vi "PH_PP_CurrentMeas_Test.vi"() -> ()   [LabVIEW 2014, in "PH_PP_CurrentMeas.lvlib"]
doc: "This VI was developed to test the PH_PPMA_DAQ RT Server Application.\n\nPlease use the PH_PPMA_DAQClient Class within the CS framework."
uses:
  PH_PP_CurrentMeas.lvlib
  PH_PP_CurrentMeas.CommandCluster.ctl
panel:
  out "Error unpacking Data? Port 6343":bool
  out "Error unpacking Data? Port 6342":bool
  out "Error unpacking Data? Port 6341":bool
  in  "Reset Error":bool
  out "6343 not connected?":bool
  out "6342 not connected?":bool
  out "6341 not connected?":bool
  out "error out":errorcluster
  in  "Tab Control":enum32{"Port 6341", "Port 6342", "Port 6343"}(tab)
  out "No Connection on 6341":bool
  out "No Data achieved due to \nno Trigger Signal on 6341":bool
  out "No Data achieved due to \nTask Failure on 6341":bool
  out "No Task defined on 6341":bool
  out "Measurement Port 6341":waveform(dbl)[](graph) caption="Measurement Data Port 6341"
  in  "Port 6341":bool
  in  "Check Port 6341":bool
  out "Received Data Sets Port 6341":T1[](array[typedef])
  out "No Connection on 6342":bool
  out "No Data achieved due to \nno Trigger Signal on 6342":bool
  out "No Data achieved due to \nTask Failure on 6342":bool
  out "No Task defined on 6342":bool
  in  "Port 6342":bool
  in  "Check Port 6342":bool
  out "Received Data Sets Port 6342":T1[](array[typedef])
  out "Measurement Port 6342":waveform(dbl)[](graph) caption="Measurement Data Port 6342"
  out "No Connection on 6343":bool
  out "No Data achieved due to \nno Trigger Signal on 6343":bool
  out "No Data achieved due to \nTask Failure on 6343":bool
  out "No Task defined on 6343":bool
  in  "Port 6343":bool
  in  "Check Port 6343":bool
  out "Received Data Sets Port 6343":T1[](array[typedef])
  out "Measurement Port 6343":waveform(dbl)[](graph) caption="Measurement Data Port 6341"
  in  "stop":bool
  in  "DAQ Server":string="phpxi001.gsi.de"
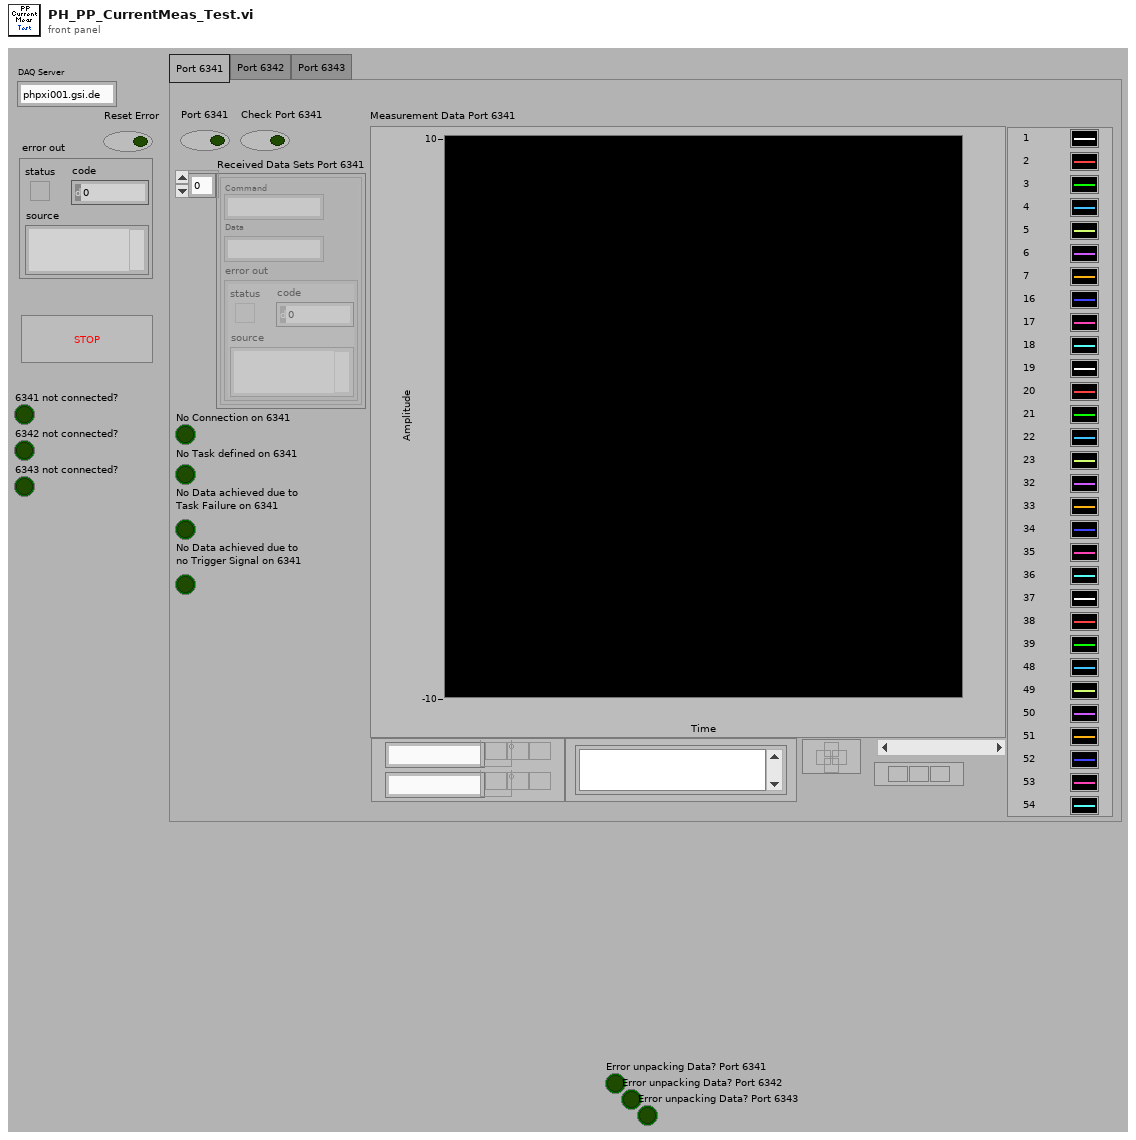
[diagram p1: front panel]
types:
  T1 = typedef "PH_PP_CurrentMeas.lvlib/PH_PP_CurrentMeas.CommandCluster.ctl" = cluster{"Command":string, "Data":string, "error out":errorcluster}
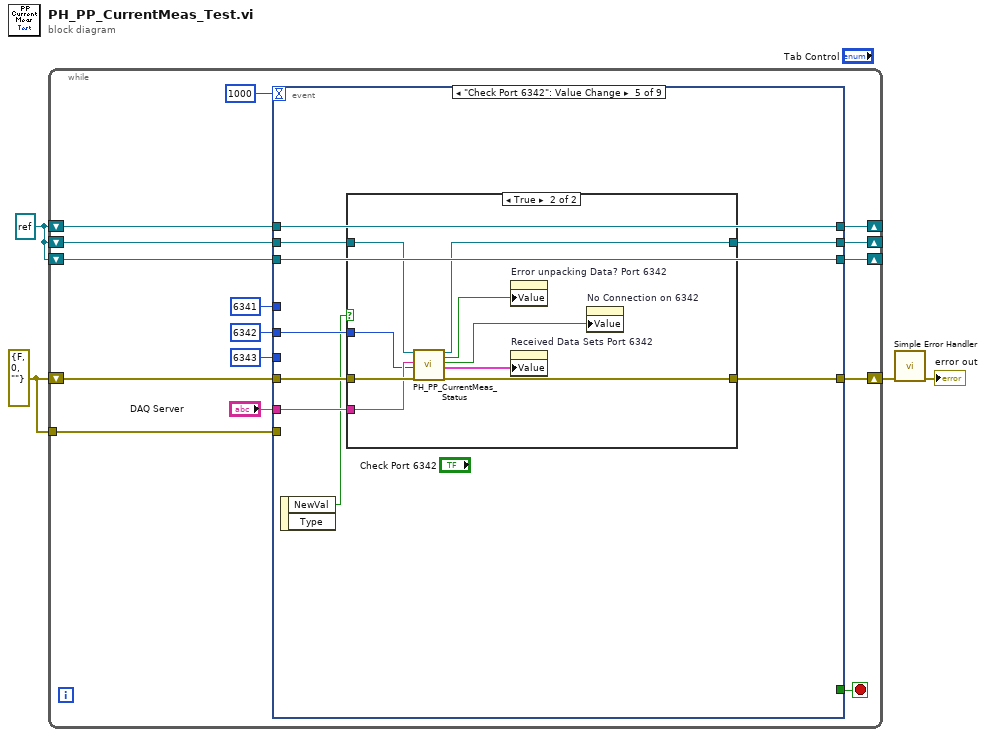
[diagram p0: block diagram]
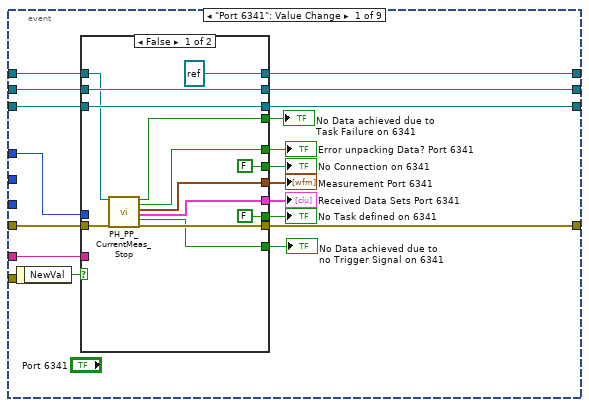
[diagram p2: hidden frame]
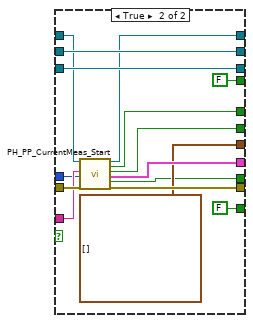
[diagram p3: hidden frame]
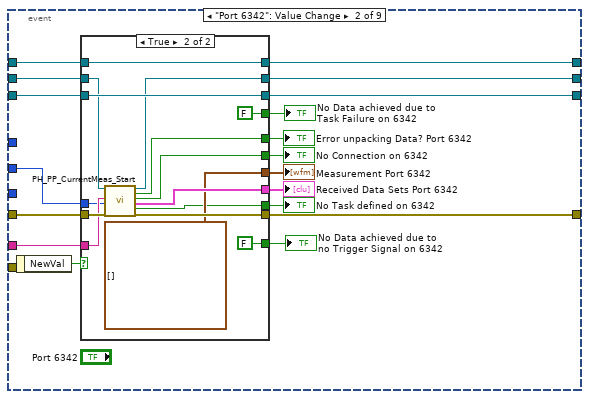
[diagram p4: hidden frame]
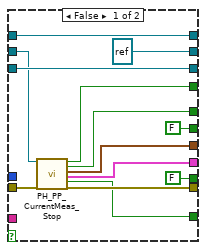
[diagram p5: hidden frame]
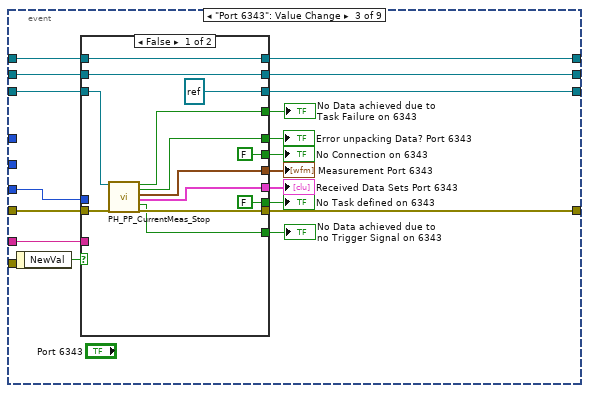
[diagram p6: hidden frame]
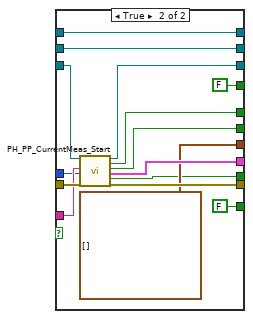
[diagram p7: hidden frame]
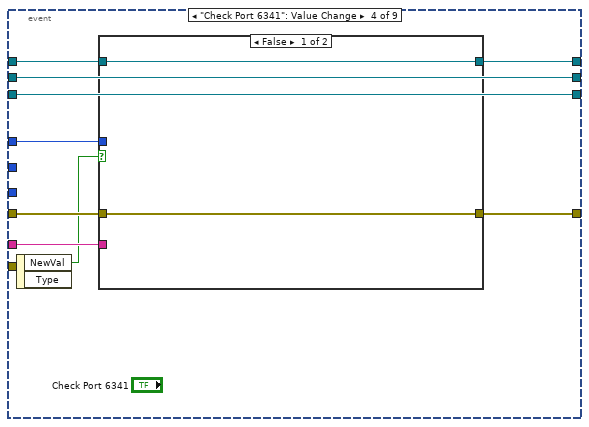
[diagram p8: hidden frame]
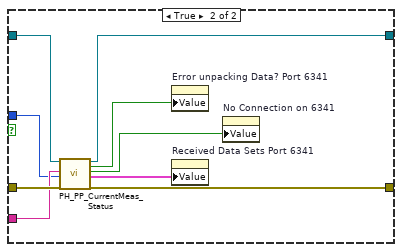
[diagram p9: hidden frame]
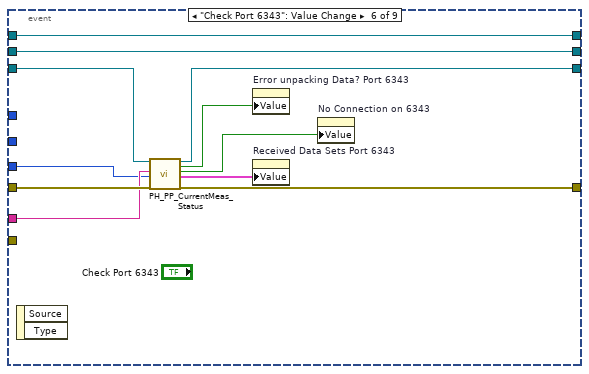
[diagram p11: hidden frame]
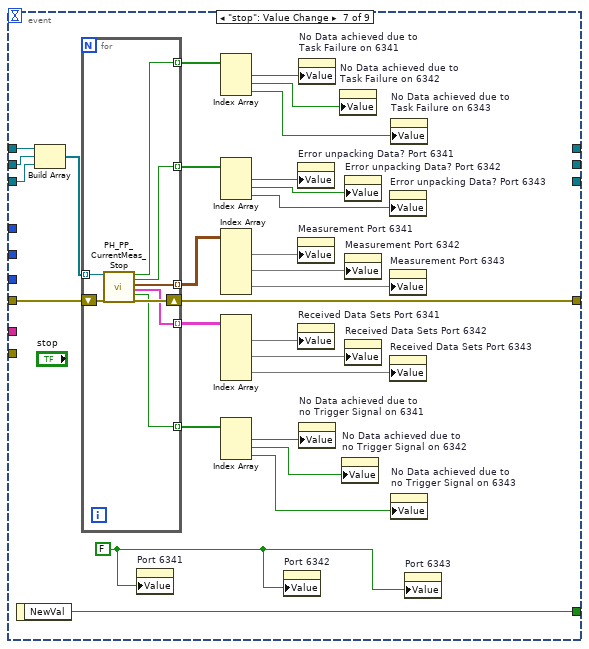
[diagram p12: hidden frame]
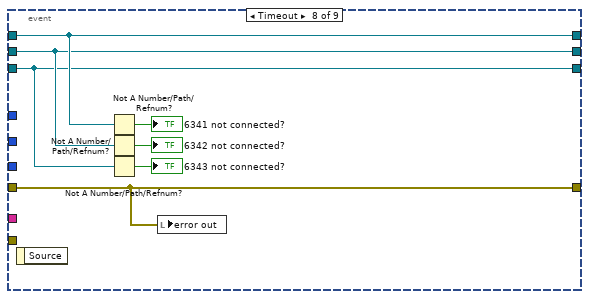
[diagram p13: hidden frame]
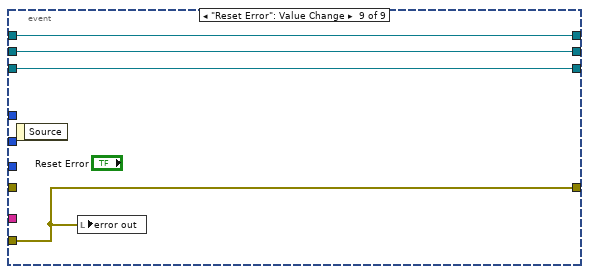
[diagram p14: hidden frame]
diagram:
  w2 = refnum<k5> refnum ("TCP Network Connection out")
  w1 = errorcluster {"status"=FALSE, "code"=0, "source"=""} ("error out")
  n1 = while {
    shift-right: [w12] -> _
    shift-left: w2 -> [w19]
    shift-right: [w16] -> w4
    shift-left: w1 -> [w18]
    shift-right: [w11] -> _
    shift-left: w2 -> [w14]
    shift-right: [w10] -> _
    shift-left: w2 -> [w13]
    tunnel: w1 -> [w5]
    stop <- w17 stop-if-true
    n2 = event shown="[4] \"Check Port 6342\": Value Change" {
      selector: _ -> [_ _ _ _ _ _ _ _ _]
      dyn-events: _ -> [_ _ _ _ _ _ _ _ _]
      timeout: 1000 -> [_ _ _ _ _ _ _ _ _]
      tunnel: w19 -> [w37 w83 w129 w164 w181 w205 w232 w248 w255]
      tunnel: [w36 w82 w128 w163 w181 w205 _ w248 w255] -> w12
      tunnel: [w28 w74 w120 w161 w184 w207 w235 w245 w252] -> w16
      tunnel: w18 -> [w31 w77 w123 w162 w185 w208 w230 w245 _]
      tunnel: [_ _ _ _ _ _ w236 _ _] -> w17
      tunnel: "DAQ Server" -> [w29 w75 w121 w160 w183 w206 _ _ _]
      tunnel: [w34 w80 w126 w166 w179 w203 _ w247 w254] -> w11
      tunnel: w14 -> [w35 w81 w127 w166 w180 w203 w234 w247 w254]
      tunnel: [w32 w78 w124 w165 w186 w201 _ w246 w253] -> w10
      tunnel: w13 -> [w33 w79 w125 w165 w186 w202 w233 w246 w253]
      tunnel: u16 6341 ("Port") -> [w27 _ _ w159 _ _ _ _ _]
      tunnel: u16 6342 ("Port") -> [_ w70 _ _ w182 _ _ _ _]
      tunnel: u16 6343 ("Port") -> [_ _ w116 _ _ w204 _ _ _]
      tunnel: w5 -> [_ _ _ _ _ _ _ _ w252]
      event "Port 6341": Value Change {
        n3 = event-data() -> ("NewVal"=w30:bool)  [unwired: 1 in]
        n4 = case shown="False" w30 {
          tunnel: [refnum<k5> refnum ("connection ID out") w59] -> w36
          tunnel: w37 -> [w46 w60]
          tunnel: [w47 w58] -> w28
          tunnel: w31 -> [w48 w63]
          tunnel: w29 -> [_ w62]
          tunnel: w35 -> [w50 w65]
          tunnel: [w50 w65] -> w34
          tunnel: [w49 w64] -> w32
          tunnel: w33 -> [w49 w64]
          tunnel: w27 -> [_ w61]
          tunnel: [w45 w56] -> w26
          tunnel: [w44 w57] -> w25
          tunnel: [w42 waveform(dbl)[] [] ("Measurement Data")] -> w24
          tunnel: [FALSE ("No Task defined?") w54] -> w23
          tunnel: [FALSE ("Connection not established") w53] -> w22
          tunnel: [w39 FALSE ("No Data achieved due to Task Failure")] -> w21
          tunnel: [w38 FALSE ("No Data achieved due to no Trigger Signal")] -> w20
          frame False {
            n5 = call "PH_PP_CurrentMeas_Stop.vi"("connection ID in"=w46, "error in (no error)"=w48) -> ("No Data achieved due to Task Failure"=w39:bool, "Error unpacking Data?"=w44:bool, "Measurement Data"=w42:waveform(dbl)[], "Receveived Data Sets"=w45:T1[], "No Data achieved due to no Trigger Signal"=w38:bool, "error out"=w47:errorcluster)  [unwired: 12 in]
          }
          frame True {
            n6 = call "PH_PP_CurrentMeas_Start.vi"("connection ID in"=w60, "NI6071E DAQ Server"=w62, "Port"=w61, "error in (no error)"=w63) -> ("connection ID out"=w59:refnum<k5>, "Error unpacking the Data?"=w57:bool, "Connection not established"=w53:bool, "Received Data Sets"=w56:T1[], "No Task defined?"=w54:bool, "error out"=w58:errorcluster)  [unwired: 10 in]
          }
        }
        "Received Data Sets Port 6341" <- w26
        "Error unpacking Data? Port 6341" <- w25
        "Measurement Port 6341" <- w24
        "No Task defined on 6341" <- w23
        "No Connection on 6341" <- w22
        "No Data achieved due to \nTask Failure on 6341" <- w21
        "No Data achieved due to \nno Trigger Signal on 6341" <- w20
      }
      event "Port 6342": Value Change {
        n7 = event-data() -> ("NewVal"=w76:bool)  [unwired: 1 in]
        n8 = case shown="True" w76 {
          tunnel: [w88 w103] -> w82
          tunnel: w83 -> [w88 w103]
          tunnel: [w94 w107] -> w74
          tunnel: w77 -> [w95 w110]
          tunnel: w75 -> [_ w109]
          tunnel: w81 -> [w89 w102]
          tunnel: [refnum<k5> refnum ("connection ID out") w101] -> w80
          tunnel: [w96 w111] -> w78
          tunnel: w79 -> [w96 w111]
          tunnel: w70 -> [_ w108]
          tunnel: [w93 w105] -> w73
          tunnel: [w92 w106] -> w72
          tunnel: [w91 waveform(dbl)[] [] ("Measurement Data")] -> w71
          tunnel: [FALSE ("No Task defined?") w100] -> w69
          tunnel: [FALSE ("Connection not established") w99] -> w68
          tunnel: [w85 FALSE ("No Data achieved due to Task Failure")] -> w67
          tunnel: [w84 FALSE ("No Data achieved due to no Trigger Signal")] -> w66
          frame False {
            n9 = call "PH_PP_CurrentMeas_Stop.vi"("connection ID in"=w89, "error in (no error)"=w95) -> ("No Data achieved due to Task Failure"=w85:bool, "Error unpacking Data?"=w92:bool, "Measurement Data"=w91:waveform(dbl)[], "Receveived Data Sets"=w93:T1[], "No Data achieved due to no Trigger Signal"=w84:bool, "error out"=w94:errorcluster)  [unwired: 12 in]
          }
          frame True {
            n10 = call "PH_PP_CurrentMeas_Start.vi"("connection ID in"=w102, "NI6071E DAQ Server"=w109, "Port"=w108, "error in (no error)"=w110) -> ("connection ID out"=w101:refnum<k5>, "Error unpacking the Data?"=w106:bool, "Connection not established"=w99:bool, "Received Data Sets"=w105:T1[], "No Task defined?"=w100:bool, "error out"=w107:errorcluster)  [unwired: 10 in]
          }
        }
        "Received Data Sets Port 6342" <- w73
        "Error unpacking Data? Port 6342" <- w72
        "Measurement Port 6342" <- w71
        "No Task defined on 6342" <- w69
        "No Connection on 6342" <- w68
        "No Data achieved due to \nTask Failure on 6342" <- w67
        "No Data achieved due to \nno Trigger Signal on 6342" <- w66
      }
      event "Port 6343": Value Change {
        n11 = event-data() -> ("NewVal"=w122:bool)  [unwired: 1 in]
        n12 = case shown="False" w122 {
          tunnel: [w137 w150] -> w128
          tunnel: w129 -> [w137 w150]
          tunnel: [w141 w154] -> w120
          tunnel: w123 -> [w142 w157]
          tunnel: w121 -> [_ w156]
          tunnel: w127 -> [w135 w149]
          tunnel: [w135 w149] -> w126
          tunnel: [refnum<k5> refnum ("connection ID out") w147] -> w124
          tunnel: w125 -> [w134 w148]
          tunnel: w116 -> [_ w155]
          tunnel: [w140 w152] -> w119
          tunnel: [w139 w153] -> w118
          tunnel: [w138 waveform(dbl)[] [] ("Measurement Data")] -> w117
          tunnel: [FALSE ("No Task defined?") w146] -> w115
          tunnel: [FALSE ("Connection not established") w145] -> w114
          tunnel: [w131 FALSE ("No Data achieved due to Task Failure")] -> w113
          tunnel: [w130 FALSE ("No Data achieved due to no Trigger Signal")] -> w112
          frame False {
            n13 = call "PH_PP_CurrentMeas_Stop.vi"("connection ID in"=w134, "error in (no error)"=w142) -> ("No Data achieved due to Task Failure"=w131:bool, "Error unpacking Data?"=w139:bool, "Measurement Data"=w138:waveform(dbl)[], "Receveived Data Sets"=w140:T1[], "No Data achieved due to no Trigger Signal"=w130:bool, "error out"=w141:errorcluster)  [unwired: 12 in]
          }
          frame True {
            n14 = call "PH_PP_CurrentMeas_Start.vi"("connection ID in"=w148, "NI6071E DAQ Server"=w156, "Port"=w155, "error in (no error)"=w157) -> ("connection ID out"=w147:refnum<k5>, "Error unpacking the Data?"=w153:bool, "Connection not established"=w145:bool, "Received Data Sets"=w152:T1[], "No Task defined?"=w146:bool, "error out"=w154:errorcluster)  [unwired: 10 in]
          }
        }
        "Received Data Sets Port 6343" <- w119
        "Error unpacking Data? Port 6343" <- w118
        "Measurement Port 6343" <- w117
        "No Task defined on 6343" <- w115
        "No Connection on 6343" <- w114
        "No Data achieved due to \nno Trigger Signal on 6343" <- w112
        "No Data achieved due to \nTask Failure on 6343" <- w113
      }
      event "Check Port 6341": Value Change {
        n15 = event-data() -> ("NewVal"=w158:bool)  [unwired: 1 in, 1 out]
        n16 = case shown="False" w158 {
          tunnel: w164 -> [w168 w177]
          tunnel: [w168 w176] -> w163
          tunnel: w162 -> [w167 w175]
          tunnel: [w167 w174] -> w161
          tunnel: w160 -> [_ w173]
          tunnel: w159 -> [_ w172]
          frame False {
          }
          frame True {
            n17 = call "PH_PP_CurrentMeas_Status.vi"("connection ID in"=w177, "NI6071E DAQ Server"=w173, "Port"=w172, "error in (no error)"=w175) -> ("connection ID out"=w176:refnum<k5>, "Error unpacking Data?"=w171:bool, "Connection not established"=w169:bool, "Receveived Data Sets"=w170:T1[], "error out"=w174:errorcluster)  [unwired: 11 in]
            n18 = property on="Error unpacking Data? Port 6341" class="Bool (strict)"("Value"=w171) -> ()  [unwired: 2 in, 2 out]
            n19 = property on="Received Data Sets Port 6341" class="Arr (strict)"("Value"=w170) -> ()  [unwired: 2 in, 2 out]
            n20 = property on="No Connection on 6341" class="Bool (strict)"("Value"=w169) -> ()  [unwired: 2 in, 2 out]
          }
        }
      }
      event "Check Port 6342": Value Change {
        n21 = event-data() -> ("NewVal"=w178:bool)  [unwired: 1 in, 1 out]
        n22 = case shown="True" w178 {
          tunnel: w185 -> [w187 w197]
          tunnel: [w187 w196] -> w184
          tunnel: w183 -> [_ w195]
          tunnel: w182 -> [_ w194]
          tunnel: w180 -> [w188 w193]
          tunnel: [w188 w192] -> w179
          frame False {
          }
          frame True {
            n23 = call "PH_PP_CurrentMeas_Status.vi"("connection ID in"=w193, "NI6071E DAQ Server"=w195, "Port"=w194, "error in (no error)"=w197) -> ("connection ID out"=w192:refnum<k5>, "Error unpacking Data?"=w190:bool, "Connection not established"=w189:bool, "Receveived Data Sets"=w191:T1[], "error out"=w196:errorcluster)  [unwired: 11 in]
            n24 = property on="Error unpacking Data? Port 6342" class="Bool (strict)"("Value"=w190) -> ()  [unwired: 2 in, 2 out]
            n25 = property on="Received Data Sets Port 6342" class="Arr (strict)"("Value"=w191) -> ()  [unwired: 2 in, 2 out]
            n26 = property on="No Connection on 6342" class="Bool (strict)"("Value"=w189) -> ()  [unwired: 2 in, 2 out]
          }
        }
      }
      event "Check Port 6343": Value Change {
        n27 = event-data() -> ()  [unwired: 1 in, 2 out]
        n28 = call "PH_PP_CurrentMeas_Status.vi"("connection ID in"=w202, "NI6071E DAQ Server"=w206, "Port"=w204, "error in (no error)"=w208) -> ("connection ID out"=w201:refnum<k5>, "Error unpacking Data?"=w200:bool, "Connection not established"=w198:bool, "Receveived Data Sets"=w199:T1[], "error out"=w207:errorcluster)  [unwired: 11 in]
        n29 = property on="Error unpacking Data? Port 6343" class="Bool (strict)"("Value"=w200) -> ()  [unwired: 2 in, 2 out]
        n30 = property on="Received Data Sets Port 6343" class="Arr (strict)"("Value"=w199) -> ()  [unwired: 2 in, 2 out]
        n31 = property on="No Connection on 6343" class="Bool (strict)"("Value"=w198) -> ()  [unwired: 2 in, 2 out]
      }
      event "stop": Value Change {
        w217 = FALSE
        n32 = event-data() -> ("NewVal"=w236:bool)  [unwired: 1 in]
        n33 = Build Array(w232, w234, w233) -> (w231:refnum<k5>[])
        n34 = for {
          shift-right: [w242] -> w235
          shift-left: w230 -> [w244]
          tunnel: w231 -> [w243] mode=indexing
          tunnel: [w239] -> w227 mode=indexing
          tunnel: [w241] -> w229 mode=indexing
          tunnel: [w240] -> w228 mode=indexing
          tunnel: [w238] -> w216 mode=indexing
          tunnel: [w237] -> w215 mode=indexing
          n35 = call "PH_PP_CurrentMeas_Stop.vi"("connection ID in"=w243, "error in (no error)"=w244) -> ("No Data achieved due to Task Failure"=w238:bool, "Error unpacking Data?"=w241:bool, "Measurement Data"=w240:waveform(dbl)[], "Receveived Data Sets"=w239:T1[], "No Data achieved due to no Trigger Signal"=w237:bool, "error out"=w242:errorcluster)  [unwired: 12 in]
        }
        n36 = property on="Port 6341" class="Bool (strict)"("Value"=w217) -> ()  [unwired: 2 in, 2 out]
        n37 = Index Array(array=w216) -> (element #1=w214:bool, element #2=w213:bool, element #3=w212:bool)  [unwired: 3 in]
        n38 = Index Array(array=w229) -> (element #1=w226:bool, element #2=w223:bool, element #3=w218:bool)  [unwired: 3 in]
        n39 = Index Array(array=w228) -> (element #1=w225:waveform(dbl)[], element #2=w222:waveform(dbl)[], element #3=w219:waveform(dbl)[])  [unwired: 6 in]
        n40 = Index Array(array=w227) -> (element #1=w224:T1[], element #2=w221:T1[], element #3=w220:T1[])  [unwired: 6 in]
        n41 = Index Array(array=w215) -> (element #1=w211:bool, element #2=w210:bool, element #3=w209:bool)  [unwired: 3 in]
        n42 = property on="Port 6342" class="Bool (strict)"("Value"=w217) -> ()  [unwired: 2 in, 2 out]
        n43 = property on="Error unpacking Data? Port 6341" class="Bool (strict)"("Value"=w226) -> ()  [unwired: 2 in, 2 out]
        n44 = property on="Measurement Port 6341" class="WFGraph (strict)"("Value"=w225) -> ()  [unwired: 2 in, 2 out]
        n45 = property on="Received Data Sets Port 6341" class="Arr (strict)"("Value"=w224) -> ()  [unwired: 2 in, 2 out]
        n46 = property on="No Data achieved due to \nTask Failure on 6341" class="Bool (strict)"("Value"=w214) -> ()  [unwired: 2 in, 2 out]
        n47 = property on="No Data achieved due to \nno Trigger Signal on 6341" class="Bool (strict)"("Value"=w211) -> ()  [unwired: 2 in, 2 out]
        n48 = property on="No Data achieved due to \nTask Failure on 6342" class="Bool (strict)"("Value"=w213) -> ()  [unwired: 2 in, 2 out]
        n49 = property on="No Data achieved due to \nno Trigger Signal on 6342" class="Bool (strict)"("Value"=w210) -> ()  [unwired: 2 in, 2 out]
        n50 = property on="Error unpacking Data? Port 6342" class="Bool (strict)"("Value"=w223) -> ()  [unwired: 2 in, 2 out]
        n51 = property on="Measurement Port 6342" class="WFGraph (strict)"("Value"=w222) -> ()  [unwired: 2 in, 2 out]
        n52 = property on="Received Data Sets Port 6342" class="Arr (strict)"("Value"=w221) -> ()  [unwired: 2 in, 2 out]
        n53 = property on="Error unpacking Data? Port 6343" class="Bool (strict)"("Value"=w218) -> ()  [unwired: 2 in, 2 out]
        n54 = property on="Measurement Port 6343" class="WFGraph (strict)"("Value"=w219) -> ()  [unwired: 2 in, 2 out]
        n55 = property on="Received Data Sets Port 6343" class="Arr (strict)"("Value"=w220) -> ()  [unwired: 2 in, 2 out]
        n56 = property on="No Data achieved due to \nTask Failure on 6343" class="Bool (strict)"("Value"=w212) -> ()  [unwired: 2 in, 2 out]
        n57 = property on="No Data achieved due to \nno Trigger Signal on 6343" class="Bool (strict)"("Value"=w209) -> ()  [unwired: 2 in, 2 out]
        n58 = property on="Port 6343" class="Bool (strict)"("Value"=w217) -> ()  [unwired: 2 in, 2 out]
      }
      event Timeout {
        n59 = event-data() -> ()  [unwired: 1 in, 1 out]
        n60 = Not A Number/Path/Refnum?(number/path/refnum=w248) -> (NaN/Path/Refnum?=→"6341 not connected?":bool)
        n61 = Not A Number/Path/Refnum?(number/path/refnum=w247) -> (NaN/Path/Refnum?=→"6342 not connected?":bool)
        n62 = Not A Number/Path/Refnum?(number/path/refnum=w246) -> (NaN/Path/Refnum?=→"6343 not connected?":bool)
        n63 = local write "error out"(w245) -> ()
      }
      event "Reset Error": Value Change {
        n64 = event-data() -> ()  [unwired: 1 in, 1 out]
        n65 = local write "error out"(w252) -> ()
      }
    }
  }
  n66 = call <vilib>:"Simple Error Handler.vi"("error in (no error)"=w4) -> ("error out"=→"error out":errorcluster)  [unwired: 4 in, 4 out]
